vi "single sweep - rus init.vi"(4 "Generate F array":bool=TRUE, 6 "Format":enum16{"Real/Imaginary", "Polar"}(ring), 7 "Setup time, s/pt":dbl=0.0001, 8 "error in (no error)":errorcluster, 9 "Lock-in DAQ settings":T7={"Lockin mode"=enum."NI-DAQ", "DAQmx Device"="Dev1", "SR Lockin"="GPIB0::10::INSTR", "Clock Multiplier"=10, "Low-pass filter"=enum."No filtering", "Ranges and couplings "=[{"Range"=1.0, "Coupling"=10106}], "Samples per read"=10, "Record IF"=FALSE, "Auto-phase"=FALSE, "RP IP Addres"="172.20.117.190"} {"Ranges and couplings"."Coupling" items=["default"=-1, "RSE"=10083, "NRSE"=10078, "Differential"=10106, "Pseudodifferential"=12529]}, 10 "Save data settings":T5={"Save data"=TRUE, "Data Root Path"=path "C:/data/RUS/RUS-YBCO-Jan2011/Sample2/Round2/singlesweep", "File Prefix"="280.36300K_1500_2500_", "File Format"=enum."ASCII", "Save column names"=TRUE, "File Comments"="<Description of the current file>", "User/Prj"="<User Name/Project Description>"}, 11 "Fast swep settings":T3={"Update rate (Hz)"=100.0, "Start F, Hz"=2000000.0, "Stop F"=3500000.0, "Number of points"=10000, "Amplitude"=2.1, "Init&amplitude"=TRUE, "IF"=1000.0, "Time constant"=0.03} {"IF" format="%#_6p"; "Amplitude" min=0.0 max=2.5; "Number of points" format="%.0p"; "Stop F" format="%#_6p"; "Start F, Hz" format="%#_6p"; "Update rate (Hz)" format="%0.2f"}) -> (0 "error out":errorcluster, 2 "Actual setup time, ms":u32=1525, 3 "RUS settings out":T1={"NI-DAQ lockin settings"={"Samples per sine wave"=0, "Sine waves per freq step"=0, "Output Representation"=enum."Real/Imaginary", "Low-pass filter"=enum."Butterworth", "Ranges and couplings "=[]}, "Fast swep settings"={"Update rate (Hz)"=250.0, "Start F, Hz"=200000.0, "Stop F"=1700000.0, "Number of points"=30000, "Amplitude"=2.1, "Init&amplitude"=TRUE, "IF"=1000.0, "Time constant"=0.1}, "Pre-sweep delay, s"=0.0, "Lockin mode"=enum."NI-DAQ", "SR Lockin"="GPIB0::10::INSTR", "DAQmx Device"="Dev3", "Clock Multiplier"=64, "Fast Sweep Data Out"={"DO clock task"="", "DO task"="", "Update clock task"="", "DAQ lockin task"="", "Pre-sweep counter task"=""}, "Lockin Range, V"=0.0, "F Array"=[], "Freq. update clock terminal"="", "DO Clock Rate (Hz)"=5000000.0, "ADC clock terminal"="/PFI4", "Pre-sweep counter terminal"="", "Samples per read"=10, "DO clock terminal"="", "Pre-sweep points"=0, "F points per write"=1000, "Total sweep time, s"=0.0, "Initial SYNTH phase"=0.0, "Record IF"=FALSE, "Save data settings"={"Save data"=TRUE, "Data Root Path"=path "", "File Prefix"="", "File Format"=enum."ASCII", "Save column names"=TRUE, "File Comments"="<Description of the current file>", "User/Prj"="<User Name/Project Description>"}, "Data file path"=path "", "New data user event"=refnum, "Stop user event"=refnum, "Number of channels"=1, "Auto-phase"=FALSE, "RP Transeiver"=refnum} {"Lockin Range, V" format="%#_6e"; "Fast swep settings"."IF" format="%#_6p"; "Fast swep settings"."Amplitude" min=0.0 max=2.5; "Fast swep settings"."Number of points" format="%.0p"; "Fast swep settings"."Stop F" format="%#_6p"; "Fast swep settings"."Start F, Hz" format="%#_6p"; "Fast swep settings"."Update rate (Hz)" format="%0.2f"; "NI-DAQ lockin settings"."Ranges and couplings"."Coupling" items=["default"=-1, "RSE"=10083, "NRSE"=10078, "Differential"=10106, "Pseudodifferential"=12529]}, 5 "Event Registration Refnum":refnum<event-registration>)   [LabVIEW 2016]
uses:
  NHMFL_Core/Libraries/Red Pitaya/RP Core/RP Transceiver/RP Transceiver.lvclass
  D:/github/NHMFL_Core/Libraries/Red Pitaya/RP Core/RP Instrument/RP Instrument.lvclass
  resonant_ultrasound/Libraries/RUS/Controls/Sweep settings.ctl
  resonant_ultrasound/Libraries/RUS/Controls/Lock-in DAQ settings.ctl
  NHMFL_Core/Libraries/File/Controls/File formats.ctl
  NHMFL_Core/Libraries/File/Controls/Save data settings.ctl
  resonant_ultrasound/Libraries/RUS/Controls/RUS NI-DAQ Lockin Settings.ctl
  resonant_ultrasound/Libraries/RUS/Controls/RUS settings.ctl
  resonant_ultrasound/Libraries/RUS/Controls/Lockin mode.ctl
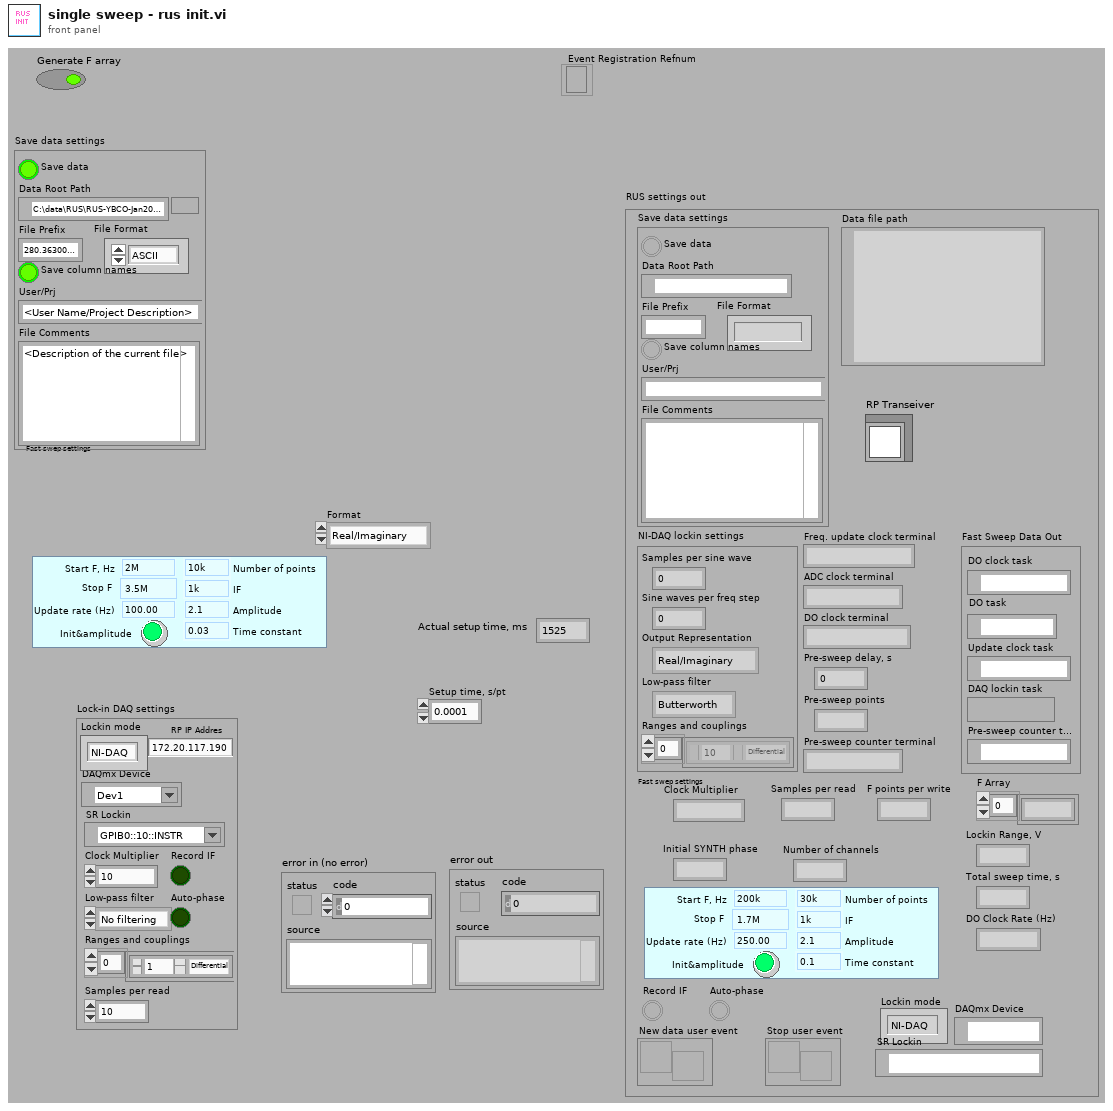
[diagram p1: front panel]
types:
  T1 = typedef "RUS settings.ctl" = cluster{"NI-DAQ lockin settings":T2, "Fast swep settings":T3, "Pre-sweep delay, s":dbl, "Lockin mode":T4, "SR Lockin":refnum<visa-resource-name>, "DAQmx Device":tag, "Clock Multiplier":i32, "Fast Sweep Data Out":cluster{"DO clock task":refnum<k21>, "DO task":refnum<k21>, "Update clock task":refnum<k21>, "DAQ lockin task":refnum<k21>, "Pre-sweep counter task":refnum<k21>}, "Lockin Range, V":sgl, "F Array":dbl[], "Freq. update clock terminal":string, "DO Clock Rate (Hz)":dbl, "ADC clock terminal":string, "Pre-sweep counter terminal":string, "Samples per read":i32, "DO clock terminal":string, "Pre-sweep points":i32, "F points per write":i32, "Total sweep time, s":dbl, "Initial SYNTH phase":dbl, "Record IF":bool, "Save data settings":T5, "Data file path":path, "New data user event":refnum<user-event>, "Stop user event":refnum<user-event>, "Number of channels":i32, "Auto-phase":bool, "RP Transeiver":refnum<class "RP Transceiver.lvclass">}
  T2 = typedef "RUS NI-DAQ Lockin Settings.ctl" = cluster{"Samples per sine wave":i32, "Sine waves per freq step":i32, "Output Representation":enum16{"Real/Imaginary", "Polar"}, "Low-pass filter":enum16{"No filtering", "Butterworth", "Bessel"}, "Ranges and couplings ":cluster{"Range":dbl, "Coupling":i32}[]}
  T3 = typedef "Sweep settings.ctl" = cluster{"Update rate (Hz)":dbl, "Start F, Hz":dbl, "Stop F":dbl, "Number of points":i32, "Amplitude":dbl, "Init&amplitude":bool, "IF":dbl, "Time constant":dbl}
  T4 = typedef "Lockin mode.ctl" = enum16{"SRS", "NI-DAQ", "Pitaya"}
  T5 = typedef "Save data settings.ctl" = cluster{"Save data":bool, "Data Root Path":path, "File Prefix":string, "File Format":T6, "Save column names":bool, "File Comments":string, "User/Prj":string}
  T6 = typedef "File formats.ctl" = enum16{"TDMS", "ASCII", "BINARY"}
  T7 = typedef "Lock-in DAQ settings.ctl" = cluster{"Lockin mode":T4, "DAQmx Device":tag, "SR Lockin":refnum<visa-resource-name>, "Clock Multiplier":i32, "Low-pass filter":enum16{"No filtering", "Butterworth", "Bessel"}, "Ranges and couplings ":cluster{"Range":dbl, "Coupling":i32}[], "Samples per read":i32, "Record IF":bool, "Auto-phase":bool, "RP IP Addres":string}
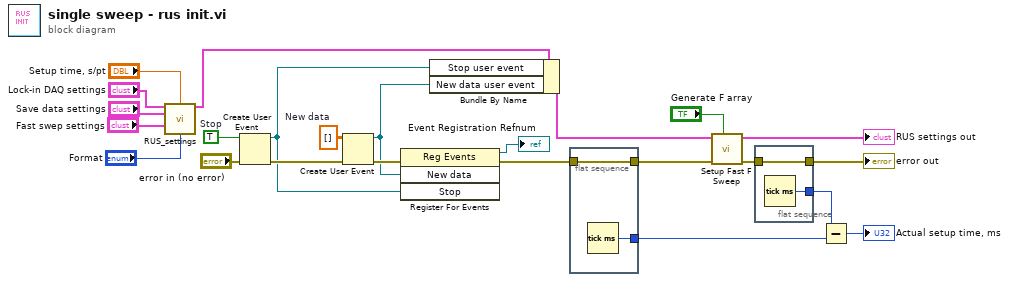
[diagram p0: block diagram]
diagram:
  w12 = TRUE  # Stop
  w9 = dbl[][] []  # New data
  n1 = call "RUS_settings.vi"("Lock-in DAQ settings"="Lock-in DAQ settings", "Setup time, s/pt"="Setup time, s/pt", "Save data settings"="Save data settings", "Fast swep settings"="Fast swep settings", "Output Representation"="Format") -> ("RUS settings"=w7:T1)  [unwired: 10 in]
  n2 = Create User Event(user event datatype=w12, error in="error in (no error)") -> (user event=w5:refnum<user-event>, error out=w11:errorcluster)
  n3 = Create User Event(user event datatype=w9, error in=w11) -> (user event=w6:refnum<user-event>, error out=w10:errorcluster)
  n4 = register-events(error in=w10, w6, w5) -> (reference out=→"Event Registration Refnum":refnum<event-registration>, error out=w3:errorcluster)  [unwired: 1 in]
  n5 = Bundle By Name(cluster=w7, "Stop user event"=w5, "New data user event"=w6) -> (w2:T1)
  n6 = flat-sequence {
    tunnel: [w26] -> w19
    tunnel: w3 -> [w25]
    tunnel: [w25] -> w22
    frame #0 {
      n7 = Tick Count (ms)() -> (millisecond timer value=w26:u32)
    }
  }
  n8 = call "Setup Fast F Sweep.vi"("Generate F array"="Generate F array", "error in"=w22, "RUS settings in"=w2) -> ("error out"=w21:errorcluster, "RUS settings out"=→"RUS settings out":T1)  [unwired: 2 in, 5 out]
  n9 = flat-sequence {
    tunnel: [w28] -> w20
    tunnel: w21 -> [w27]
    tunnel: [w27] -> w13
    frame #0 {
      n10 = Tick Count (ms)() -> (millisecond timer value=w28:u32)
    }
  }
  n11 = Subtract(x=w20, y=w19) -> (x-y=→"Actual setup time, ms":u32)
  "error out" <- w13
